vi "CIMAQ_Skeleton.vi"(8 "error in (no error)":errorcluster, 11 "Refnum in":T1) -> (0 "error out":errorcluster, 3 "Refnum out":T1)   [LabVIEW 2017]
uses:
  <vilib>/vision/Image Controls.llb/IMAQ Image.ctl
  <vilib>/vision/NI_Vision_Development_Module.lvlib
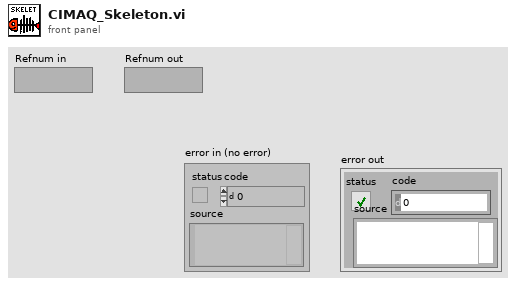
[diagram p1: front panel]
types:
  T1 = typedef "IMAQ Image.ctl" = refnum<image>
  T2 = typedef "Image Type" = u32
  T3 = enum32{"AutoM", "Close", "Dilate", "Erode", "Gradient", "Gradient out", "Gradient in", "Hit miss", "Open", "PClose", "POpen", "Thick", "Thin"}
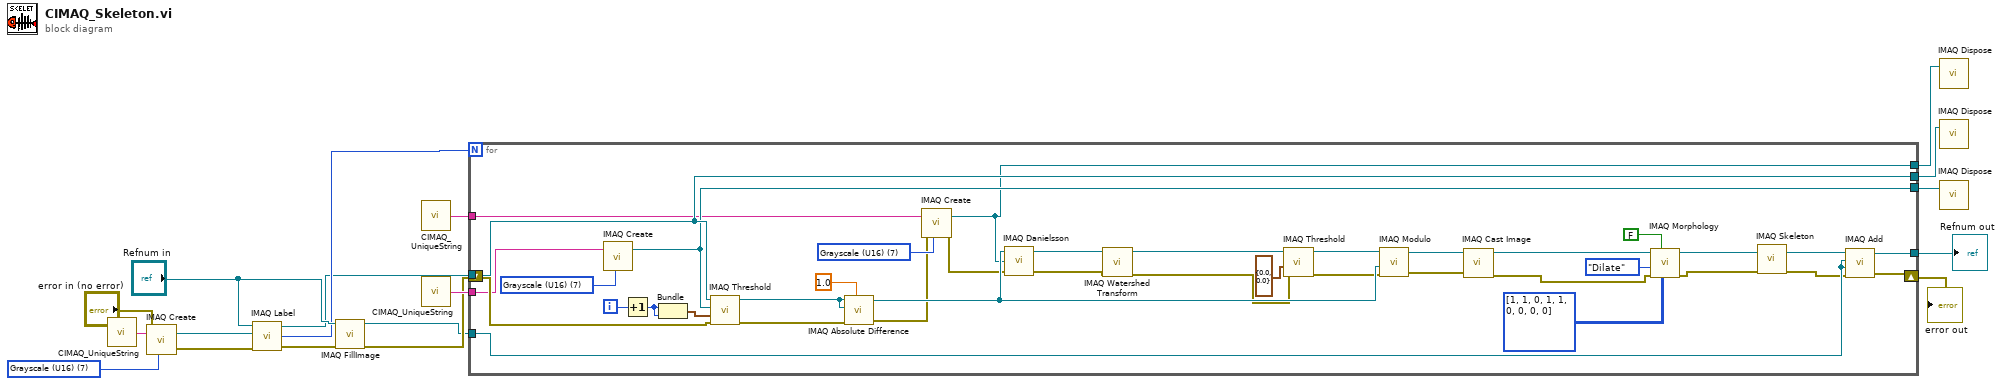
[diagram p0: block diagram]
diagram:
  w12 = T2 7 items=["Grayscale (U8)", "Grayscale (I16)", "Grayscale (SGL)", "Complex (CSG)", "RGB (U32)", "HSL (U32)", "RGB (U64)", "Grayscale (U16)"] ("Image Type")
  n1 = call <userlib>:"CIMAQ_UniqueString.vi"() -> ("String"=w4:string)  [unwired: 5 in]
  n2 = call "IMAQ Create"("Image Name"=w4, "Image Type"=w12, "error in (no error)"="error in (no error)") -> ("New Image"=w5:T1, "error out"=w2:errorcluster)  [unwired: 2 in]
  n3 = call "IMAQ Label"("error in (no error)"=w2, "Image Dst"=w5, "Image Src"="Refnum in") -> ("error out"=w8:errorcluster, "Number of Particles"=w10:i32, "Image Dst Out"=w6:T1)  [unwired: 1 in]
  n4 = call "IMAQ FillImage"("error in (no error)"=w8, "Image"="Refnum in") -> ("error out"=w11:errorcluster, "Image Out"=w9:T1)  [unwired: 8 in]
  n5 = call <userlib>:"CIMAQ_UniqueString.vi"() -> ("String"=w16:string)  [unwired: 5 in]
  n6 = call <userlib>:"CIMAQ_UniqueString.vi"() -> ("String"=w14:string)  [unwired: 5 in]
  n7 = for {
    N: w10 -> [_]
    tunnel: w6 -> [w52]
    tunnel: [w52] -> w7
    tunnel: w9 -> [w51]
    tunnel: [w49] -> w13
    tunnel: w14 -> [w47]
    tunnel: [w46] -> w15
    tunnel: w16 -> [w44]
    tunnel: [w35] -> w17
    shift-right: [w19] -> w3
    shift-left: w11 -> [w54]
    i -> [w56]
    w48 = T2 7 items=["Grayscale (U8)", "Grayscale (I16)", "Grayscale (SGL)", "Complex (CSG)", "RGB (U32)", "HSL (U32)", "RGB (U64)", "Grayscale (U16)"] ("Image Type")
    w50 = T2 7 items=["Grayscale (U8)", "Grayscale (I16)", "Grayscale (SGL)", "Complex (CSG)", "RGB (U32)", "HSL (U32)", "RGB (U64)", "Grayscale (U16)"] ("Image Type")
    n8 = call "IMAQ Create"("Image Name"=w47, "Image Type"=w50) -> ("New Image"=w46:T1)  [unwired: 3 in, 1 out]
    n9 = Increment(x=w56) -> (x+1=w55:i32)
    n10 = Bundle(w55, w55) -> (w53:cluster{i32, i32})  [unwired: 1 in]
    n11 = call "IMAQ Threshold"("error in (no error)"=w54, "Range"=w53, "Image Dst"=w46, "Image Src"=w52) -> ("error out"=w29:errorcluster, "Image Dst Out"=w39:T1)  [unwired: 6 in]
    n12 = call "IMAQ Absolute Difference"("Image Src A"=w39, "Constant"=1.0, "Image Dst"=w39, "error in (no error)"=w29) -> ("Image Dst Out"=w37:T1, "error out"=w28:errorcluster)  [unwired: 3 in]
    n13 = call "IMAQ Create"("Image Name"=w44, "Image Type"=w48, "error in (no error)"=w28) -> ("New Image"=w35:T1, "error out"=w27:errorcluster)  [unwired: 2 in]
    n14 = call "IMAQ Danielsson"("error in (no error)"=w27, "Image Dst"=w35, "Image Src"=w37) -> ("error out"=w26:errorcluster, "Image Dst Out"=w43:T1)  [unwired: 1 in]
    n15 = call "IMAQ Watershed Transform"("error in (no error)"=w26, "Image Src"=w43) -> ("error out"=w25:errorcluster, "Image Dst Out"=w42:T1)  [unwired: 7 in, 1 out]
    n16 = call "IMAQ Threshold"("error in (no error)"=w25, "Range"=cluster{"Lower value":sgl, "Upper value":sgl} {"Lower value"=0.0, "Upper value"=0.0}, "Image Src"=w42) -> ("error out"=w24:errorcluster, "Image Dst Out"=w36:T1)  [unwired: 7 in]
    n17 = call "IMAQ Modulo"("Image Src A"=w36, "Image Src B"=w37, "error in (no error)"=w24) -> ("Image Dst Out"=w40:T1, "error out"=w23:errorcluster)  [unwired: 4 in]
    n18 = call "IMAQ Cast Image"("error in (no error)"=w23, "Image Src"=w40) -> ("error out"=w22:errorcluster, "Image Dst Out"=w38:T1)  [unwired: 8 in]
    n19 = call "IMAQ Morphology"("Structuring Element"=i32[][] [[1, 1, 0], [1, 1, 0], [0, 0, 0]], "Square/Hexa (Square)"=FALSE, "error in (no error)"=w22, "Operation"=T3."Dilate", "Image Src"=w38) -> ("error out"=w21:errorcluster, "Image Dst Out"=w34:T1)  [unwired: 5 in]
    n20 = call "IMAQ Skeleton"("error in (no error)"=w21, "Image Src"=w34) -> ("error out"=w20:errorcluster, "Image Dst Out"=w30:T1)  [unwired: 4 in]
    n21 = call "IMAQ Add"("Image Src A"=w30, "Image Dst"=w51, "Image Src B"=w51, "error in (no error)"=w20) -> ("Image Dst Out"=w49:T1, "error out"=w19:errorcluster)  [unwired: 3 in]
  }
  "Refnum out" <- w13
  "error out" <- w3
  n22 = call "IMAQ Dispose"("Image"=w17) -> ()  [unwired: 5 in, 1 out]
  n23 = call "IMAQ Dispose"("Image"=w7) -> ()  [unwired: 5 in, 1 out]
  n24 = call "IMAQ Dispose"("Image"=w15) -> ()  [unwired: 5 in, 1 out]
